vi "Display Item in Tree.vi"(4 "Condensed?":bool=TRUE, 5 "Item Name":string, 7 "Parent Tag":string, 8 "error in (no error)":errorcluster, 10 "Data":variant, 11 "Tree Refnum":refnum<vi>) -> (0 "error out":errorcluster, 3 "Tree Refnum out":refnum<vi>)   [LabVIEW 2015, in "YAML Parser.lvclass"]
uses:
  YAML Parser.lvclass
  <vilib>/ErrorRing/Error Ring.xnode
  <vilib>/Utility/Data Type/NI_Data Type.lvlib
  YAML Parser.lvlib
  <vilib>/Utility/error.llb/whitespace.ctl
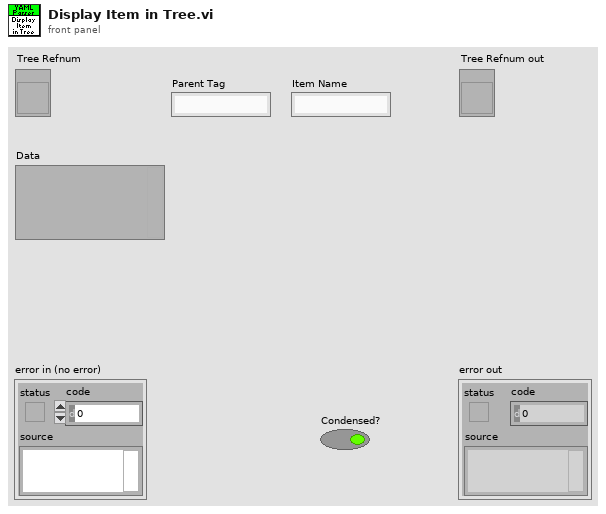
[diagram p1: front panel]
types:
  T1 = typedef "NI_Data Type.lvlib/Data Type.ctl" = enum8{"Invalid Type", "Void", "I8", "I16", "I32", "I64", "U8", "U16", "U32", "U64", "Single Float", "Double Float", "Extended Float", "Single Complex", "Double Complex", "Extended Complex", "Enum U8", "Enum U16", "Enum U32", "Enum U64", "Single Float With Unit", "Double Float With Unit", "Extended Float With Unit", "Single Complex with Unit", "Double Complex with Unit", "Extended Complex with Unit", "Boolean", "String", "Path", "Picture", "Tag", "Array", "Cluster", "Variant", "LV Variant", "Waveform", "Timestamp", "Digital Waveform", "Digital Data", "ExpressData", "Refnum", "External Data", "VI", "Poly VI", "LabVIEW Class Instance", "Fixed Point"}
  T2 = typedef "whitespace.ctl" = u16
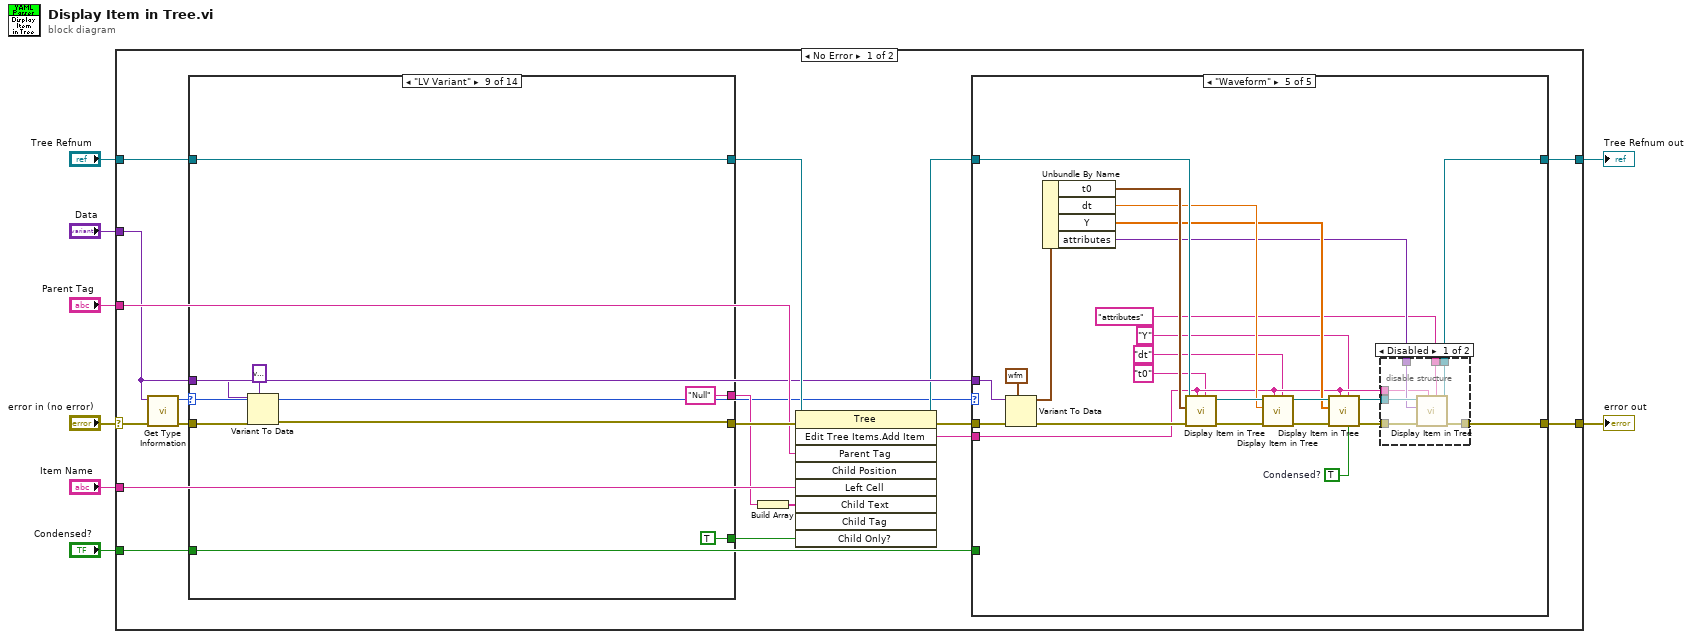
[diagram p0: block diagram]
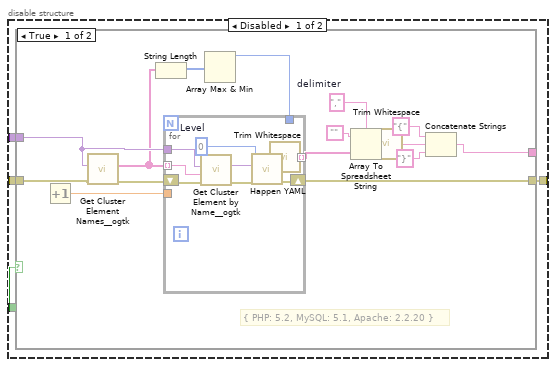
[diagram p4: hidden frame]
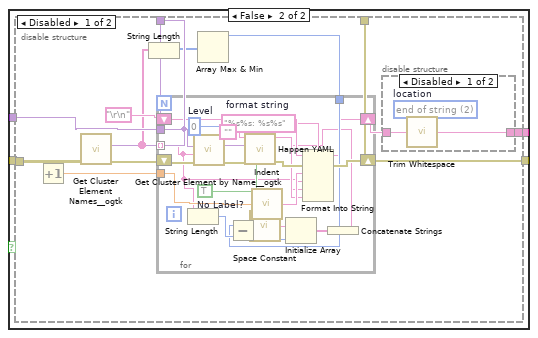
[diagram p5: hidden frame]
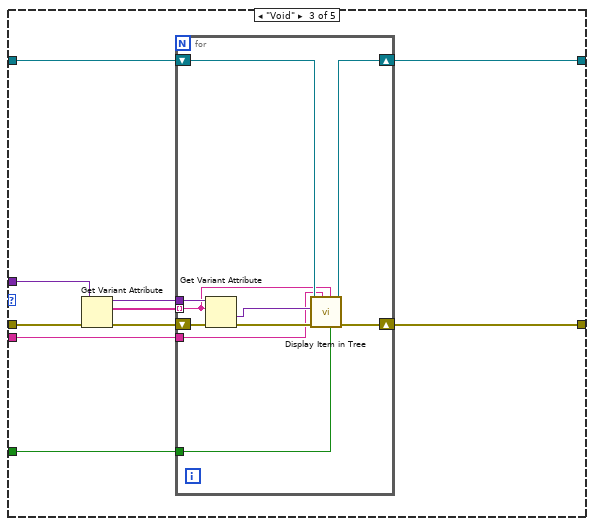
[diagram p8: hidden frame]
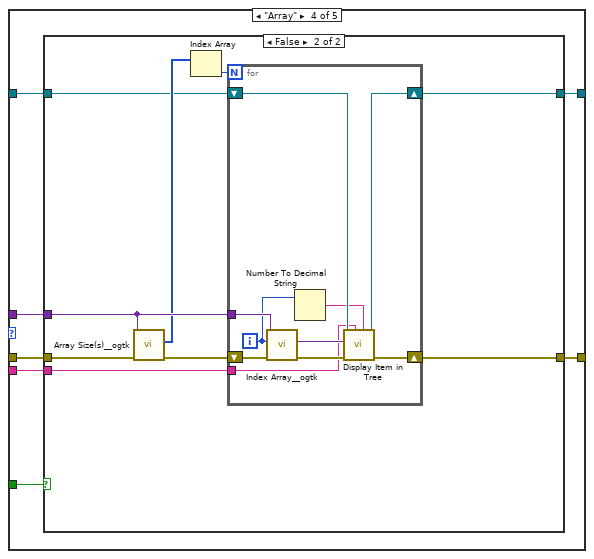
[diagram p9: hidden frame]
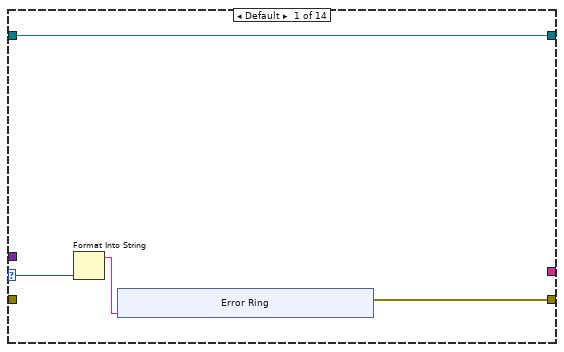
[diagram p12: hidden frame]
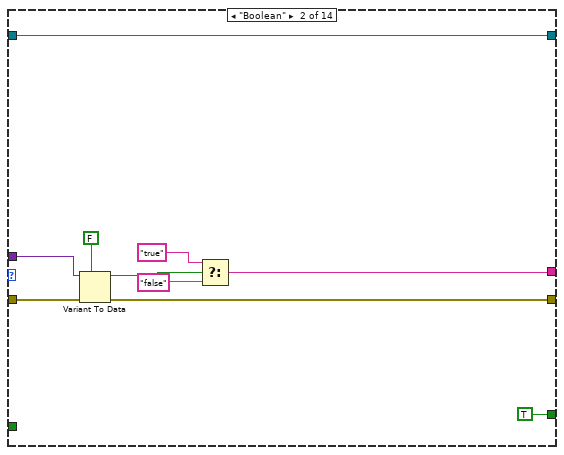
[diagram p13: hidden frame]
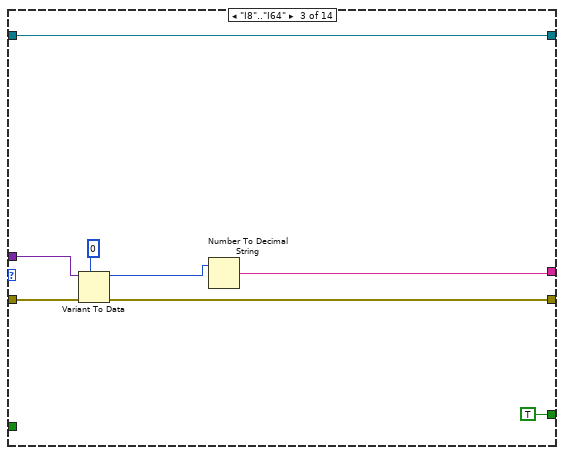
[diagram p14: hidden frame]
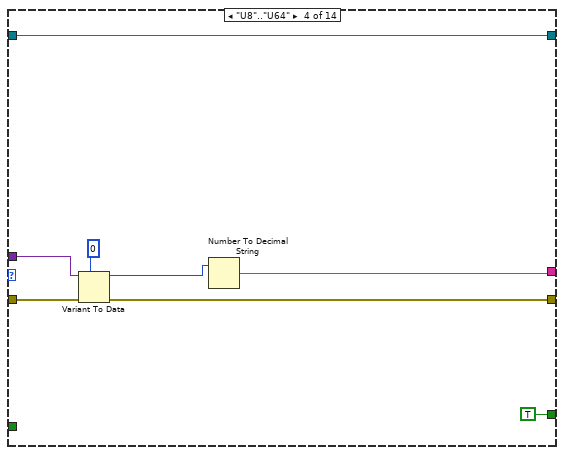
[diagram p15: hidden frame]
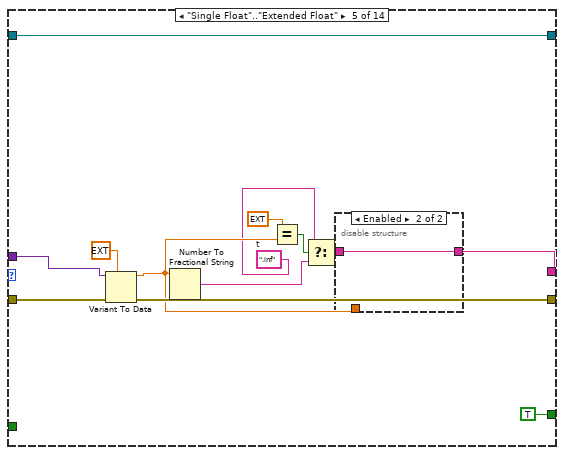
[diagram p16: hidden frame]
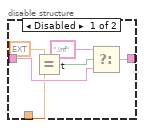
[diagram p17: hidden frame]
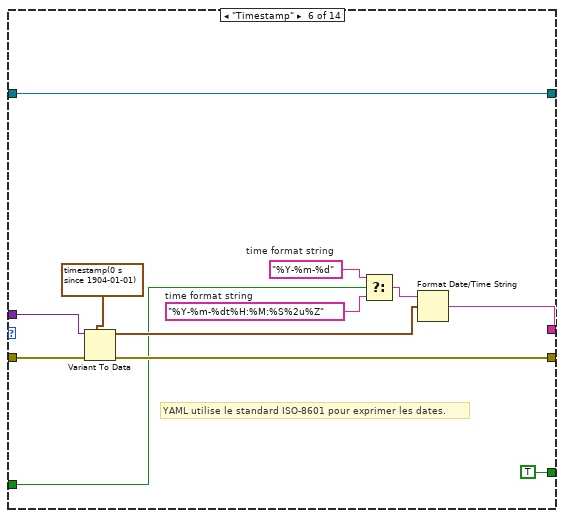
[diagram p18: hidden frame]
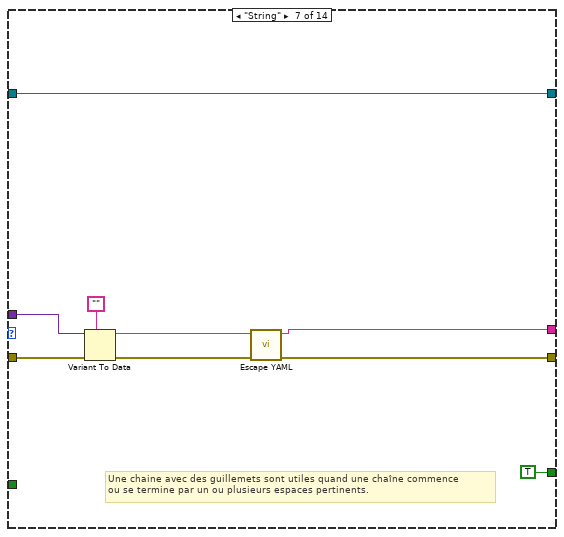
[diagram p19: hidden frame]
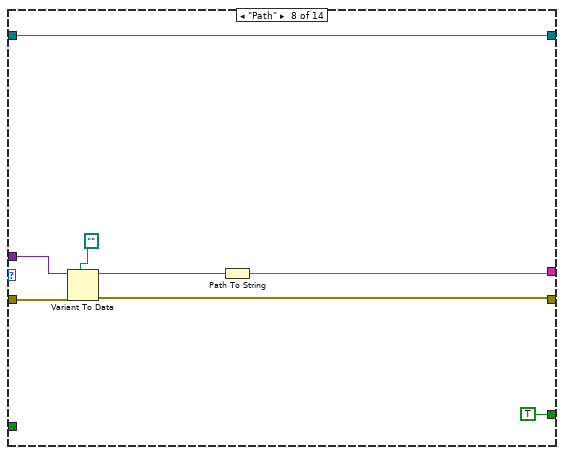
[diagram p20: hidden frame]
diagram:
  n1 = case shown="No Error" "error in (no error)" {
    selector: "error in (no error)" -> [w26 w332]
    tunnel: [w15 w332] -> w7
    tunnel: [w11 w331] -> w4
    tunnel: "Tree Refnum" -> [w20 w331]
    tunnel: "Condensed?" -> [w9 _]
    tunnel: "Data" -> [w13 _]
    tunnel: "Parent Tag" -> [w23 _]
    tunnel: "Item Name" -> [w19 _]
    frame No Error {
      n2 = call <vilib>:"Get Type Information.vi"("error in (no error)"=w26, "Variant"=w13) -> ("error out"=w25:errorcluster, "Type"=w10:T1)  [unwired: 5 in, 3 out]
      n3 = case shown="\"LV Variant\"" w10 {
        selector: w10 -> [w186 _ _ _ _ _ _ _ _ _ _ _ _ _]
        tunnel: w25 -> [_ w204 w212 w220 w233 w252 w260 w269 w276 w278 w283 w291 w300 w304]
        tunnel: w13 -> [_ w203 w211 w219 w232 w251 w259 w268 w275 _ w282 w290 _ w302]
        tunnel: [w187 w201 w209 w217 w230 w248 w256 w264 w273 w278 w280 w289 w300 w303] -> w24
        tunnel: [_ w197 w207 w215 w223 w247 w255 w265 "Null" ("YAML String") w277 w281 _ _ w301] -> w18
        tunnel: w9 -> [_ _ _ _ _ w246 _ _ _ _ _ _ _ w305]
        tunnel: [_ TRUE TRUE TRUE TRUE TRUE TRUE TRUE TRUE _ _ _ _ _] -> w22
        tunnel: [w189 w195 w205 w213 w221 w241 w253 w262 w271 w279 w288 w292 w299 w306] -> w21
        tunnel: w20 -> [w189 w195 w205 w213 w221 w241 w253 w262 w271 w279 w288 w292 w299 w306]
        frame Default {
          n4 = Format Into String(w186) -> (resulting string=w188:string)  [unwired: 3 in, 1 out]
          n5 = xnode "Error Ring"("parameter 0"=w188) -> ("error out"=w187:errorcluster)
        }
        frame "Boolean" {
          n6 = Variant To Data(error in=w204, type=FALSE, Variant=w203) -> (data=w200:bool, error out=w201:errorcluster)
          n7 = Select(t="true", s=w200, f="false") -> (s? t:f=w197:string)
        }
        frame "I8".."I64" {
          n8 = Variant To Data(error in=w212, type=i64 0, Variant=w211) -> (data=w208:i64, error out=w209:errorcluster)
          n9 = Number To Decimal String(number=w208) -> (decimal integer string=w207:string)  [unwired: 1 in]
        }
        frame "U8".."U64" {
          n10 = Variant To Data(error in=w220, type=u64 0, Variant=w219) -> (data=w216:u64, error out=w217:errorcluster)
          n11 = Number To Decimal String(number=w216) -> (decimal integer string=w215:string)  [unwired: 1 in]
        }
        frame "Single Float".."Extended Float" {
          w224 = ".inf"  # t
          n12 = Variant To Data(error in=w233, type=ext 0.0, Variant=w232) -> (data=w225:ext, error out=w230:errorcluster)
          n13 = Number To Fractional String(number=w225) -> (F-format string=w227:string)  [unwired: 3 in]
          n14 = Equal?(x=ext inf, y=w225) -> (x = y?=w228:bool)
          n15 = Select(t=w224, s=w228, f=w227) -> (s? t:f=w226:string)
          n16 = disable-structure shown="Enabled" {
            disable-tunnel: w226 -> [w237 w240]
            disable-tunnel: w225 -> [w236 _]
            disable-tunnel: [w234 w240] -> w223
            frame Disabled {
              w235 = ".inf"  # t
              n17 = Equal?(x=ext -inf, y=w236) -> (x = y?=w238:bool)
              n18 = Select(t=w235, s=w238, f=w237) -> (s? t:f=w234:string)
            }
            frame Enabled {
            }
          }
        }
        frame "Timestamp" {
          w244 = "%Y-%m-%d"  # time format string
          w245 = "%Y-%m-%dt%H:%M:%S%2u%Z"  # time format string
          # "YAML utilise le standard ISO-8601 pour exprimer les dates."
          n19 = Variant To Data(error in=w252, type=timestamp(0 s since 1904-01-01), Variant=w251) -> (data=w249:timestamp, error out=w248:errorcluster)
          n20 = Select(t=w244, s=w246, f=w245) -> (s? t:f=w243:string)
          n21 = Format Date/Time String(time format string (%c)=w243, seconds (now)=w249) -> (date/time string=w247:string)  [unwired: 1 in]
        }
        frame "String" {
          # "Une chaine avec des guillemets sont utiles quand une chaîne commence \nou se termine par un ou plusieurs espaces pertinents."
          n22 = Variant To Data(error in=w260, type="", Variant=w259) -> (data=w258:string, error out=w257:errorcluster)
          n23 = call "Escape YAML.vi"("error in (no error)"=w257, "String"=w258) -> ("error out"=w256:errorcluster, "YAML String"=w255:string)  [unwired: 8 in]
        }
        frame "Path" {
          n24 = Variant To Data(error in=w269, type=path "", Variant=w268) -> (data=w266:path, error out=w264:errorcluster)
          n25 = Path To String(path=w266) -> (string=w265:string)
        }
        frame "LV Variant" {
          n26 = Variant To Data(error in=w276, type=variant, Variant=w275) -> (error out=w273:errorcluster)  [unwired: 1 out]
        }
        frame "LabVIEW Class Instance" {
          w277 = "(binary)"  # YAML String
        }
        frame "Refnum" {
          n27 = Variant To Data(error in=w283, type=refnum<k0> refnum, Variant=w282) -> (data=w285:refnum<k0>, error out=w280:errorcluster)
          n28 = Type Cast(type=u32 0, x=w285) -> (*(type *) &x=w284:u32)
          n29 = Number To Decimal String(number=w284) -> (decimal integer string=w281:string)  [unwired: 1 in]
        }
        frame "Waveform" {
          n30 = disable-structure shown="Disabled" {
            disable-tunnel: w291 -> [w297 w298]
            disable-tunnel: w290 -> [w296 _]
            disable-tunnel: [w293 w298] -> w289
            frame Disabled {
              # "#ToCode\nRécupérer le nom de la waveform."
              n31 = Variant To Data(error in=w297, type=waveform(dbl) {"t0"=timestamp(0 s since 1904-01-01), "dt"=1.0, "Y"=[]} ("Waveform"), Variant=w296) -> (data=w294:waveform(dbl), error out=w293:errorcluster)
              n32 = Unbundle By Name(w294) -> ()  [unwired: 1 out]
            }
            frame Enabled {
            }
          }
        }
        frame "Void", "Cluster" {
        }
        frame "Array" {
          n33 = case shown="True" w305 {
            tunnel: w304 -> [w307 w314]
            tunnel: [w307 w311] -> w303
            tunnel: w302 -> [_ w313]
            tunnel: [_ w310] -> w301
            frame False {
            }
            frame True {
              w309 = "[%s]"  # format string
              w317 = ","  # delimiter
              n34 = call <userlib>:"Array Size(s)__ogtk.vi"("error in (no error)"=w314, "Array"=w313) -> ("error out"=w319:errorcluster, "Size(s)"=w321:u32[])  [unwired: 7 in, 1 out]
              n35 = Index Array(array=w321) -> (element=w320:u32)  [unwired: 1 in]
              n36 = for {
                N: w320 -> [_]
                shift-right: [w325] -> w312
                shift-left: w319 -> [w330]
                tunnel: w313 -> [w329]
                tunnel: [w327] -> w318 mode=indexing
                i -> [w328]
                w322 = TRUE  # No Label?
                n37 = call <userlib>:"Index Array__ogtk.vi"("error in (no error)"=w330, "Index (1D)"=w328, "MultiD Array"=w329) -> ("error out"=w326:errorcluster, "Array Element"=w324:variant)  [unwired: 7 in]
                n38 = call "Flatten to YAML.vi"("No Label?"=w322, "error in (no error)"=w326, "Anything"=w324) -> ("error out"=w325:errorcluster, "YAML String"=w323:string)  [unwired: 7 in]
                n39 = call <vilib>:"Trim Whitespace.vi"("string"=w323) -> ("trimmed string"=w327:string)  [unwired: 1 in]
              }
              n40 = Array To Spreadsheet String(delimiter (Tab)=w317, array=w318, 3:"") -> (spreadsheet string=w316:string)
              n41 = call <vilib>:"Trim Whitespace.vi"("string"=w316) -> ("trimmed string"=w308:string)  [unwired: 1 in]
              n42 = Format Into String(format string=w309, error in=w312, w308) -> (resulting string=w310:string, error out=w311:errorcluster)  [unwired: 1 in]
            }
          }
        }
      }
      n43 = Build Array(w18) -> (w17:string[])
      n44 = invoke class="Tree" method="Edit Tree Items.Add Item"(reference=w21, error in=w24, "Parent Tag"=w23, "Left Cell"=w19, "Child Text"=w17, "Child Only?"=w22) -> (reference out=w12:refnum<vi>, error out=w16:errorcluster, "Edit Tree Items:Add Item"=w14:string)  [unwired: 3 in, 6 out]
      n45 = case shown="\"Waveform\"" w10 {
        tunnel: w16 -> [w27 w32 w113 w130 w168]
        tunnel: w13 -> [_ w31 w112 w129 w167]
        tunnel: [w27 w33 w114 w131 w163] -> w15
        tunnel: w9 -> [_ w30 w111 w128 _]
        tunnel: [w28 w29 w109 w127 w164] -> w11
        tunnel: w12 -> [w28 w29 w110 w126 w165]
        tunnel: w14 -> [_ _ w108 w125 w158]
        frame Default {
        }
        frame "Cluster" {
          n46 = disable-structure shown="Enabled" {
            disable-tunnel: [w37 w104] -> w33
            disable-tunnel: w32 -> [w36 w104]
            disable-tunnel: w31 -> [w35 _]
            disable-tunnel: w30 -> [w34 _]
            frame Disabled {
              n47 = case shown="True" w34 {
                tunnel: [w53 w66] -> w37
                tunnel: w36 -> [w51 w65]
                tunnel: w35 -> [w49 w64]
                tunnel: [w39 w63] -> _
                frame True {
                  w45 = ","  # delimiter
                  # "{ PHP: 5.2, MySQL: 5.1, Apache: 2.2.20 }"
                  n48 = Increment() -> (x+1=w52:dbl)  [unwired: 1 in]
                  n49 = call <userlib>:"Get Cluster Element Names__ogtk.vi"("error in (no error)"=w51, "Cluster"=w49) -> ("error out"=w50:errorcluster, "Element Names"=w48:string[])  [unwired: 8 in]
                  n50 = String Length(string=w48) -> (length=w47:i32[])
                  n51 = Array Max & Min(array=w47) -> (max value=w46:i32)  [unwired: 3 out]
                  n52 = for {
                    shift-right: [w55] -> w53
                    shift-left: w50 -> [w62]
                    tunnel: w52 -> [_]
                    tunnel: w48 -> [w58] mode=indexing
                    tunnel: w49 -> [w61]
                    tunnel: w46 -> [_]
                    tunnel: [w54] -> w41 mode=indexing
                    w57 = u32 0  # Level
                    n53 = call <userlib>:"Get Cluster Element by Name__ogtk.vi"("error in (no error)"=w62, "Element Name"=w58, "Cluster"=w61) -> ("error out"=w60:errorcluster, "VElement"=w59:variant)  [unwired: 6 in, 1 out]
                    n54 = call "Happen YAML.vi"("error in (no error)"=w60, "Level"=w57, "Anything"=w59) -> ("error out"=w55:errorcluster, "YAML String out"=w56:string)  [unwired: 7 in]
                    n55 = call <vilib>:"Trim Whitespace.vi"("string"=w56) -> ("trimmed string"=w54:string)  [unwired: 1 in]
                  }
                  n56 = Array To Spreadsheet String(delimiter (Tab)=w45, array=w41, 3:"") -> (spreadsheet string=w44:string)
                  n57 = call <vilib>:"Trim Whitespace.vi"("string"=w44) -> ("trimmed string"=w38:string)  [unwired: 1 in]
                  n58 = Concatenate Strings("{", w38, "}") -> (w39:string)
                }
                frame False {
                  n59 = disable-structure shown="Disabled" {
                    disable-tunnel: [w77 _] -> w66
                    disable-tunnel: w65 -> [w73 _]
                    disable-tunnel: w64 -> [w71 _]
                    disable-tunnel: [w70 _] -> w63
                    frame Disabled {
                      n60 = Increment() -> (x+1=w74:dbl)  [unwired: 1 in]
                      n61 = call <userlib>:"Get Cluster Element Names__ogtk.vi"("error in (no error)"=w73, "Cluster"=w71) -> ("error out"=w72:errorcluster, "Element Names"=w69:string[])  [unwired: 8 in]
                      n62 = String Length(string=w69) -> (length=w68:i32[])
                      n63 = Array Max & Min(array=w68) -> (max value=w67:i32)  [unwired: 3 out]
                      n64 = for {
                        shift-right: [w97] -> w77
                        shift-left: w72 -> [w103]
                        shift-right: [w83] -> w75
                        shift-left: "\r\n" -> [w96]
                        tunnel: w74 -> [w94]
                        tunnel: w69 -> [w90] mode=indexing
                        tunnel: w71 -> [w102]
                        tunnel: w67 -> [w88]
                        w82 = u32 0  # Level
                        w93 = "%s%s: %s%s"  # format string
                        w99 = TRUE  # No Label?
                        n65 = String Length(string=w90) -> (length=w89:i32)
                        n66 = call <userlib>:"Get Cluster Element by Name__ogtk.vi"("error in (no error)"=w103, "Element Name"=w90, "Cluster"=w102) -> ("error out"=w101:errorcluster, "VElement"=w100:variant)  [unwired: 6 in, 1 out]
                        n67 = Subtract(x=w88, y=w89) -> (x-y=w85:i32)
                        n68 = call "Happen YAML.vi"("No Label?"=w99, "error in (no error)"=w101, "Level"=w82, "Anything"=w100, "YAML String in"="") -> ("error out"=w98:errorcluster, "YAML String out"=w91:string)  [unwired: 5 in]
                        n69 = call <vilib>:"Space Constant.vi"() -> ("String"=w87:string)
                        n70 = call "Indent.vi"("Index"=w94) -> ("Indentation"=w92:string)
                        n71 = Initialize Array(w87, w85) -> (w86:string[])
                        n72 = Concatenate Strings(w86) -> (w84:string)
                        n73 = Format Into String(format string=w93, initial string=w96, error in=w98, w92, w90, w84, w91) -> (resulting string=w83:string, error out=w97:errorcluster)
                      }
                      n74 = disable-structure shown="Disabled" {
                        disable-tunnel: w75 -> [w80 w81]
                        disable-tunnel: [w79 w81] -> w70
                        frame Disabled {
                          w78 = T2 2 items=["both", "start of string", "end of string"]  # location
                          n75 = call <vilib>:"Trim Whitespace.vi"("string"=w80, "location (both)"=w78) -> ("trimmed string"=w79:string)
                        }
                        frame Enabled {
                        }
                      }
                    }
                    frame Enabled {
                    }
                  }
                }
              }
            }
            frame Enabled {
            }
          }
        }
        frame "Void" {
          n76 = Get Variant Attribute(Variant=w112, error in=w113) -> (duplicate Variant=w105:variant, names=w106:string[], error out=w107:errorcluster)  [unwired: 2 in, 1 out]
          n77 = for {
            shift-right: [w121] -> w114
            shift-left: w107 -> [w123]
            tunnel: w106 -> [w115] mode=indexing
            tunnel: w105 -> [w124]
            tunnel: w111 -> [w120]
            shift-right: [w118] -> w109
            shift-left: w110 -> [w119]
            tunnel: w108 -> [w116]
            n78 = Get Variant Attribute(Variant=w124, name=w115, error in=w123) -> (value=w117:variant, error out=w122:errorcluster)  [unwired: 1 in, 2 out]
            n79 = call "Display Item in Tree.vi"("Condensed?"=w120, "Item Name"=w115, "Parent Tag"=w116, "error in (no error)"=w122, "Data"=w117, "Tree Refnum"=w119) -> ("error out"=w121:errorcluster, "Tree Refnum out"=w118:refnum<vi>)  [unwired: 4 in]
          }
        }
        frame "Array" {
          n80 = case shown="False" w128 {
            tunnel: [w132 w142] -> w131
            tunnel: w130 -> [w132 w141]
            tunnel: w129 -> [_ w140]
            tunnel: [w133 w135] -> w127
            tunnel: w126 -> [w133 w136]
            tunnel: w125 -> [_ w134]
            frame True {
            }
            frame False {
              n81 = call <userlib>:"Array Size(s)__ogtk.vi"("error in (no error)"=w141, "Array"=w140) -> ("error out"=w137:errorcluster, "Size(s)"=w139:u32[])  [unwired: 7 in, 1 out]
              n82 = Index Array(array=w139) -> (element=w138:u32)  [unwired: 1 in]
              n83 = for {
                N: w138 -> [_]
                shift-right: [w147] -> w142
                shift-left: w137 -> [w152]
                tunnel: w140 -> [w151]
                shift-right: [w148] -> w135
                shift-left: w136 -> [w150]
                tunnel: w134 -> [w145]
                i -> [w144]
                n84 = call <userlib>:"Index Array__ogtk.vi"("error in (no error)"=w152, "Index (1D)"=w144, "MultiD Array"=w151) -> ("error out"=w149:errorcluster, "Array Element"=w146:variant)  [unwired: 7 in]
                n85 = Number To Decimal String(number=w144) -> (decimal integer string=w143:string)  [unwired: 1 in]
                n86 = call "Display Item in Tree.vi"("Item Name"=w143, "Parent Tag"=w145, "error in (no error)"=w149, "Data"=w146, "Tree Refnum"=w150) -> ("error out"=w147:errorcluster, "Tree Refnum out"=w148:refnum<vi>)  [unwired: 5 in]
              }
            }
          }
        }
        frame "Waveform" {
          w153 = TRUE  # Condensed?
          n87 = Variant To Data(error in=w168, type=waveform(dbl) {"t0"=timestamp(0 s since 1904-01-01), "dt"=1.0, "Y"=[]} ("Waveform"), Variant=w167) -> (data=w170:waveform(dbl), error out=w166:errorcluster)
          n88 = Unbundle By Name(w170) -> ("t0"=w162:timestamp, "dt"=w161:dbl, "Y"=w160:dbl[], "attributes"=w159:variant)
          n89 = call "Display Item in Tree.vi"("Item Name"="t0", "Parent Tag"=w158, "error in (no error)"=w166, "Data"=w162, "Tree Refnum"=w165) -> ("error out"=w175:errorcluster, "Tree Refnum out"=w176:refnum<vi>)  [unwired: 5 in]
          n90 = call "Display Item in Tree.vi"("Item Name"="dt", "Parent Tag"=w158, "error in (no error)"=w175, "Data"=w161, "Tree Refnum"=w176) -> ("error out"=w173:errorcluster, "Tree Refnum out"=w174:refnum<vi>)  [unwired: 5 in]
          n91 = call "Display Item in Tree.vi"("Condensed?"=w153, "Item Name"="Y", "Parent Tag"=w158, "error in (no error)"=w173, "Data"=w160, "Tree Refnum"=w174) -> ("error out"=w171:errorcluster, "Tree Refnum out"=w172:refnum<vi>)  [unwired: 4 in]
          n92 = disable-structure shown="Disabled" {
            disable-tunnel: w172 -> [w183 w185]
            disable-tunnel: w171 -> [w182 w184]
            disable-tunnel: [w181 w185] -> w164
            disable-tunnel: [w180 w184] -> w163
            disable-tunnel: w159 -> [w179 _]
            disable-tunnel: w158 -> [w178 _]
            disable-tunnel: "attributes" ("Item Name") -> [w177 _]
            frame Disabled {
              n93 = call "Display Item in Tree.vi"("Item Name"=w177, "Parent Tag"=w178, "error in (no error)"=w182, "Data"=w179, "Tree Refnum"=w183) -> ("error out"=w180:errorcluster, "Tree Refnum out"=w181:refnum<vi>)  [unwired: 5 in]
            }
            frame Enabled {
            }
          }
        }
      }
    }
    frame Error {
    }
  }
  "error out" <- w7
  "Tree Refnum out" <- w4
